vi "Camera Constants.vi"() -> (1 "fps robot":i32, 2 "compression robot":i32, 3 "img size robot":T1=enum."320x240", 4 "score limits":T2={"Rect Coverage"=76.0, "Aspect Ratio"=0.0, "X Edge Strength"=40.0, "Y Edge Strength"=50.0}, 6 "color":bool, 8 "cam type":enum16{"206", "1011"}(ring), 10 "particle count limit":i32=8, 12 "fps dashboard":i32, 13 "compression dashboard":i32, 14 "img size dashboard":T1=enum."320x240", 15 "area size limit":i32=444)   [LabVIEW 2011]
uses:
  <vilib>/Rock Robotics/WPI/Camera/WPI_CameraImageSize.ctl
panel:
  in  "Area Size Limit":i32=444
  in  "Particle Count Limit":i32=8
  in  "Score Limits":T2={"Rect Coverage"=69.0, "Aspect Ratio"=0.0, "X Edge Strength"=40.0, "Y Edge Strength"=60.0}
  in  "input cam type":enum16{"206", "1011"}(ring)
  in  "input color":bool
  in  "img size dashboard":T1=enum."320x240"
  in  "img size robot":T1=enum."320x240"
  in  "compression_dashboard":i32=40
  in  "compression_robot":i32=40
  in  "fps_dashboard":i32=20
  in  "fps_robot":i32=5
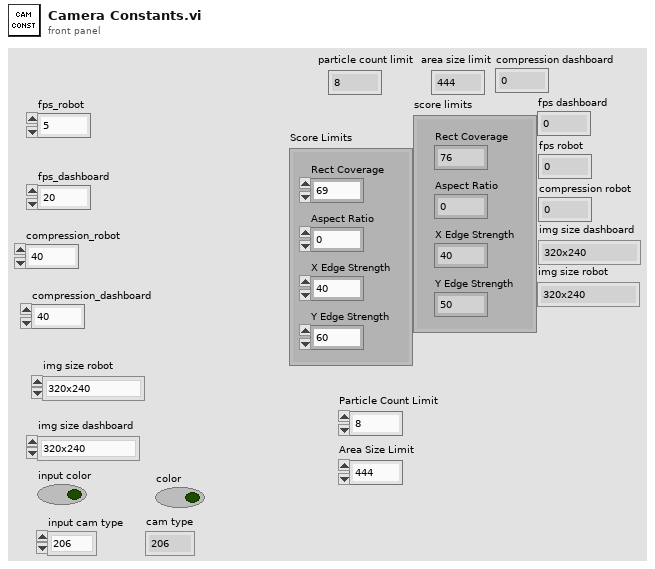
[diagram p1: front panel]
types:
  T1 = typedef "WPI_CameraImageSize.ctl" = enum16{"640x480", "320x240", "160x120"}
  T2 = cluster{"Rect Coverage":dbl, "Aspect Ratio":dbl, "X Edge Strength":dbl, "Y Edge Strength":dbl}
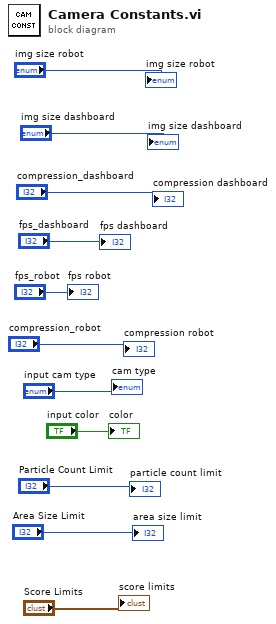
[diagram p0: block diagram]
diagram:
  "color" <- "input color"
  "cam type" <- "input cam type"
  "particle count limit" <- "Particle Count Limit"
  "area size limit" <- "Area Size Limit"
  "score limits" <- "Score Limits"
  "compression dashboard" <- "compression_dashboard"
  "fps dashboard" <- "fps_dashboard"
  "fps robot" <- "fps_robot"
  "compression robot" <- "compression_robot"
  "img size dashboard" <- "img size dashboard"
  "img size robot" <- "img size robot"
